vi "ELVIS III v1.0 Reserve Encoder.vi"(7 "Allow multiple opens?":bool, 8 "error in (no error)":errorcluster, 10 "Encoder Channel":T2, 11 "myRIO FPGA Ref Out":T1) -> (0 "error out":errorcluster)   [LabVIEW 2021]
uses:
  <vilib>/myRIO/Common/Instrument Driver Framework/myRIO v1.0/Encoder/typedefs/Encoder Channels Enum.ctl
  <vilib>/myRIO/Common/Instrument Driver Framework/Utilities/typedefs/Generic FPGA Reference.ctl
  <vilib>/myRIO/Common/Instrument Driver Framework/ELVIS III v1.0/Resource Manager/vis/ELVIS III v1.0 Create Configuration List.vi
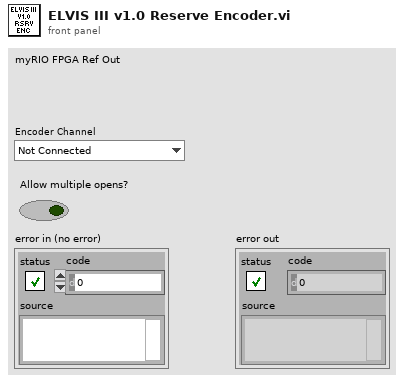
[diagram p1: front panel]
types:
  T1 = typedef "Generic FPGA Reference.ctl" = refnum<k20>
  T2 = typedef "Encoder Channels Enum.ctl" = enum16{"Not Connected", "C/ENC0", "C/ENC1", "A/ENC", "A/ENC0", "A/ENC1", "A/ENC2", "A/ENC3", "A/ENC4", "A/ENC5", "A/ENC6", "A/ENC7", "A/ENC8", "A/ENC9", "B/ENC", "B/ENC0", "B/ENC1", "B/ENC2", "B/ENC3", "B/ENC4", "B/ENC5", "B/ENC6", "B/ENC7", "B/ENC8", "B/ENC9", "DIO/ENC0", "DIO/ENC1", "DIO/ENC2", "DIO/ENC3", "DIO/ENC4"}
  T3 = typedef "ELVIS III v1.0 Channel Reservation List.ctl" = T4[]
  T4 = typedef "ELVIS III v1.0 Channel Reservation Info.ctl" = cluster{"Channel Name":string, "Connector":T5, "MutexIDs":u32[]}
  T5 = typedef "ELVIS III v1.0 Connector List.ctl" = enum32{"None", "ConnectorA", "ConnectorB"}
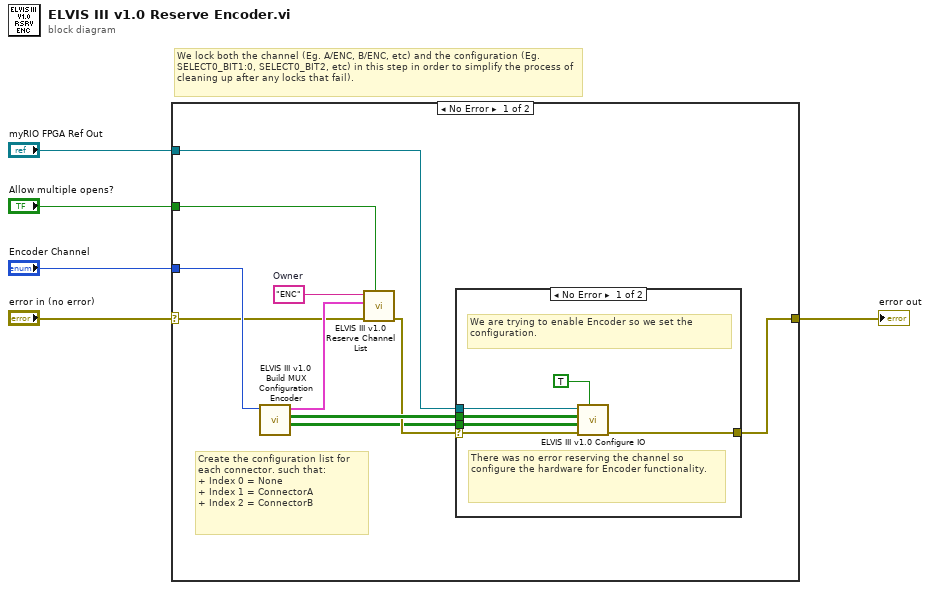
[diagram p0: block diagram]
diagram:
  # "We lock both the channel (Eg. A/ENC, B/ENC, etc) and the configuration (Eg. SELECT0_BIT1:0, SELECT0_BIT2, etc) in this step in order to simplify the process of cleaning up after any locks that fail)."
  n1 = case shown="No Error" "error in (no error)" {
    selector: "error in (no error)" -> [w10 w23]
    tunnel: "myRIO FPGA Ref Out" -> [w13 _]
    tunnel: "Encoder Channel" -> [w15 _]
    tunnel: [w7 w23] -> w3
    tunnel: "Allow multiple opens?" -> [w14 _]
    frame No Error {
      w11 = "ENC"  # Owner
      # "Create the configuration list for each connector. such that:\n+ Index 0 = None\n+ Index 1 = ConnectorA\n+ Index 2 = ConnectorB"
      n2 = call <vilib>:"ELVIS III v1.0 Build MUX Configuration Encoder.vi"("Channel"=w15) -> ("Configuration Bitmask Array"=w6:bool[][], "Configuration BitCode Array"=w9:bool[][], "Channel Reservation List"=w12:T3)  [unwired: 8 in]
      n3 = call <vilib>:"ELVIS III v1.0 Reserve Channel List.vi"("Allow multiple opens?"=w14, "error in (no error)"=w10, "Channel Reservation List"=w12, "Owner"=w11) -> ("error out"=w8:errorcluster)  [unwired: 7 in]
      n4 = case shown="No Error" w8 {
        selector: w8 -> [w18 w22]
        tunnel: w13 -> [w21 _]
        tunnel: w9 -> [w19 _]
        tunnel: [w17 w22] -> w7
        tunnel: w6 -> [w16 _]
        frame No Error {
          # "There was no error reserving the channel so configure the hardware for Encoder functionality."
          # "We are trying to enable Encoder so we set the configuration."
          n5 = call <vilib>:"ELVIS III v1.0 Configure IO.vi"("Value"=TRUE ("Clear?"), "error in (no error)"=w18, "Bitmask Array"=w16, "Bitcode Array"=w19, "myRIO FPGA Ref In"=w21) -> ("error out"=w17:errorcluster)  [unwired: 6 in]
        }
        frame Error {
        }
      }
    }
    frame Error {
      # "Nothing to do since there is an incoming error."
    }
  }
  "error out" <- w3
